vi "Launch OSK.vi"(8 "error in (no error)":errorcluster) -> (0 "error out":errorcluster)   [LabVIEW 2015, in "Win32 Util.lvlib"]
uses:
  LabSDL2/Source/Libraries/Win32 Util/Win32 Util.lvlib
  kernel32.dll
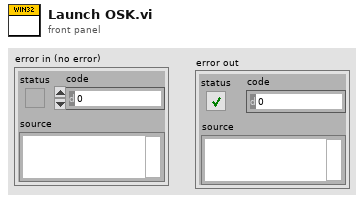
[diagram p1: front panel]
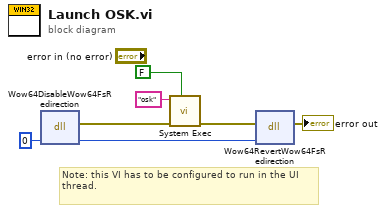
[diagram p0: block diagram]
diagram:
  # "Note: this VI has to be configured to run in the UI thread."
  n1 = dll-call lib="kernel32.dll" fn="Wow64DisableWow64FsRedirection"("OldValue"=0) -> (error out=w5:errorcluster, "OldValue"=w3:i32)  [unwired: 4 in, 1 out]
  n2 = call <vilib>:"System Exec.vi"("wait until completion? (T)"=FALSE, "error in (no error)"=w5, "command line"="osk") -> ("error out"=w4:errorcluster)  [unwired: 5 in, 3 out]
  n3 = dll-call lib="kernel32.dll" fn="Wow64RevertWow64FsRedirection"(error in=w4, "OldValue"=w3) -> (error out=→"error out":errorcluster)  [unwired: 4 in, 1 out]
